vi "path steer2.vi"(11 "lane":bool) -> (3 "handle":dbl=5.200000000000001)   [LabVIEW 2015]
uses:
  G_ALL.vi
panel:
  in  "x 3":dbl=50.0 format="%#_13g"
  in  "x 2":dbl=5.0 format="%#_13g"
  in  "x":dbl=0.2 format="%#_13g"
  out "current idx":i32=9112
  out "map_track sel":dbl[][](array[numeric])
  out "dist sel":dbl[](array[numeric])
  in  "y":dbl=0.7
  in  "y 3":dbl=6.0 format="%#_13g"
  in  "y 2":dbl=15.0 format="%#_13g"
  out "element":dbl=-42.73390488941538
  out "XY Graph":cluster{"Y":dbl[], "Y":dbl[]}[](graph)=[{"Y"=[-62.270788198222405, -61.3028587435479, -60.64797168770746, -60.00414081408834, -59.35624672898274, -58.704182799096586, -58.062869555030055, -57.324417698249775, -56.3593175353864, -55.392505243639526, -54.74987553944367, -54.107360311157855, -53.4625281010745, -52.815268660483156, -51.84490266882976, -51.19638678084248, -50.22569981527318, -49.58323485281044, -48.93987198407685, -47.97817047579251, -47.33548315463016, -46.59804499224549, -45.95694180099581, -45.31659197029625, -44.3487464210446, -43.69981062781701, -42.73390488941538, -42.082599966834195, -41.437244759678, -40.79791938631003, -40.15638313566361, -39.5161574223998, -38.23493066806538, -37.59359481763489, -36.95200424827834, -36.31462462205997, -35.66938436512903, -34.97187443953064, -34.00375998116469, -33.361996827642564, -32.72011649020922, -31.762676240541964, -31.1267605203253, -30.48871011333479, -29.53221842324259, -28.8954579631871, -28.254818864117063, -27.61302081515921, -26.651631628034465, -25.91417367981147, -24.952481253026605, -24.309631425841772, -23.676791629873463], "Y"=[206.05300612625732, 206.20998608028694, 206.31731108964544, 206.4238193812488, 206.5319939554686, 206.64187408533144, 206.75094671337308, 206.84947177394332, 207.01722005802338, 207.18752464015114, 207.30187909576753, 207.4172264991964, 207.5340024404453, 207.6519836568955, 207.83122212678202, 207.95212683530963, 208.13494101670534, 208.25718613007166, 208.38030959441758, 208.56619920738456, 208.6915241088362, 208.80142519721795, 208.92844487701353, 209.05595576734015, 209.25069887260085, 209.3822220550732, 209.5796218846342, 209.7138886173675, 209.84754269369316, 209.98075087695668, 210.11518464043854, 210.24985120575727, 210.52176541203883, 210.65907131753448, 210.79696807600604, 210.9346992584219, 211.07492355438725, 211.2107438653489, 211.4245125721372, 211.5671731458532, 211.71064662911698, 211.92621966104974, 212.0703122033147, 212.2156875009412, 212.4352208971859, 212.58227341216255, 212.73101817081624, 212.88079472174562, 213.10672138794857, 213.28129607537733, 213.51073950832134, 213.66518203900827, 213.81774856058888]}, {"Y"=array[360 elements], "Y"=array[360 elements]}]
  out "map_track":dbl[][](array[numeric])=[[-62.270788198222405, 206.05300612625732], [-61.3028587435479, 206.20998608028694], [-60.64797168770746, 206.31731108964544], [-60.00414081408834, 206.4238193812488], [-59.35624672898274, 206.5319939554686], [-58.704182799096586, 206.64187408533144], [-58.062869555030055, 206.75094671337308], [-57.324417698249775, 206.84947177394332], [-56.3593175353864, 207.01722005802338], [-55.392505243639526, 207.18752464015114], [-54.74987553944367, 207.30187909576753], [-54.107360311157855, 207.4172264991964], [-53.4625281010745, 207.5340024404453], [-52.815268660483156, 207.6519836568955], [-51.84490266882976, 207.83122212678202], [-51.19638678084248, 207.95212683530963], [-50.22569981527318, 208.13494101670534], [-49.58323485281044, 208.25718613007166], [-48.93987198407685, 208.38030959441758], [-47.97817047579251, 208.56619920738456], [-47.33548315463016, 208.6915241088362], [-46.59804499224549, 208.80142519721795], [-45.95694180099581, 208.92844487701353], [-45.31659197029625, 209.05595576734015], [-44.3487464210446, 209.25069887260085], [-43.69981062781701, 209.3822220550732], [-42.73390488941538, 209.5796218846342], [-42.082599966834195, 209.7138886173675], [-41.437244759678, 209.84754269369316], [-40.79791938631003, 209.98075087695668], [-40.15638313566361, 210.11518464043854], [-39.5161574223998, 210.24985120575727], [-38.23493066806538, 210.52176541203883], [-37.59359481763489, 210.65907131753448], [-36.95200424827834, 210.79696807600604], [-36.31462462205997, 210.9346992584219], [-35.66938436512903, 211.07492355438725], [-34.97187443953064, 211.2107438653489], [-34.00375998116469, 211.4245125721372], [-33.361996827642564, 211.5671731458532], [-32.72011649020922, 211.71064662911698], [-31.762676240541964, 211.92621966104974], [-31.1267605203253, 212.0703122033147], [-30.48871011333479, 212.2156875009412], [-29.53221842324259, 212.4352208971859], [-28.8954579631871, 212.58227341216255], [-28.254818864117063, 212.73101817081624], [-27.61302081515921, 212.88079472174562], [-26.651631628034465, 213.10672138794857], [-25.91417367981147, 213.28129607537733], [-24.952481253026605, 213.51073950832134], [-24.309631425841772, 213.66518203900827], [-23.676791629873463, 213.81774856058888]]
  out "dist":dbl[](array[numeric])=[-20.832094988384732, -19.8553041899657, -18.874727759944605, -18.211104588592054, -17.558523398263937, -16.901660791573594, -16.240403646752558, -15.589881152775536, -14.844885627682299, -13.865315410117493, -12.883618074822659, -12.2308931111174, -11.578106130467432, -10.922785445885511, -10.264861171497461, -9.27808025010812, -8.61839031874266, -7.630638219294179, -6.976646555922144, -6.3216082606081, -5.342105968983386, -4.687313388290825, -3.941730869406446, -3.2881657992313187, -2.635243956437811, -1.648000377451759, -0.9858704723425199, 1.324050382980464, 1.977105781207095, 2.6325759923136727, 3.286811460402093, 4.596574542690249, 5.252443877774635, 5.9086861917571, 6.560777187390371, 7.221078514277543, 7.931688993516377, 8.923123643119611, 9.580551954444903, 10.238271505592612, 11.219680474262686, 11.871716872015202, 12.526119117620228, 13.507481061647026, 14.16100101214439, 14.81868137409002, 15.477724430966466, 16.465303302609627, 17.22314269645568, 18.211826980021506, 18.87296871643959, 19.523939338549425, 20.177455296801384]
  out "weight":dbl[](array[numeric])=[0.0, 0.0, 0.0, 0.0, 0.0, 0.0, 0.0, 0.0, 0.0, 0.0, 0.0, 0.0, 0.0, 0.0, 0.0, 0.0, 0.0, 0.0, 0.0, 0.0, 0.0, 0.0, 0.0, 0.0, 0.0, 0.0, 0.0, 0.006618568895935004, 0.022925143850115227, 0.045607515278417665, 0.07608403237613132, 0.16836029257577229, 0.23176392233689572, 0.30677978733130234, 0.39181799555917685, 0.48644996623238884, 0.5939963001932036, 0.7424840008349528, 0.8317946790700433, 0.9072191609257558, 0.9789386113637093, 0.9976924878056614, 1.0, 1.0, 1.0, 1.0, 1.0, 1.0, 1.0, 0.9944116041666606, 0.9486136733425102, 0.8544723463308531, 0.7254699057656591]
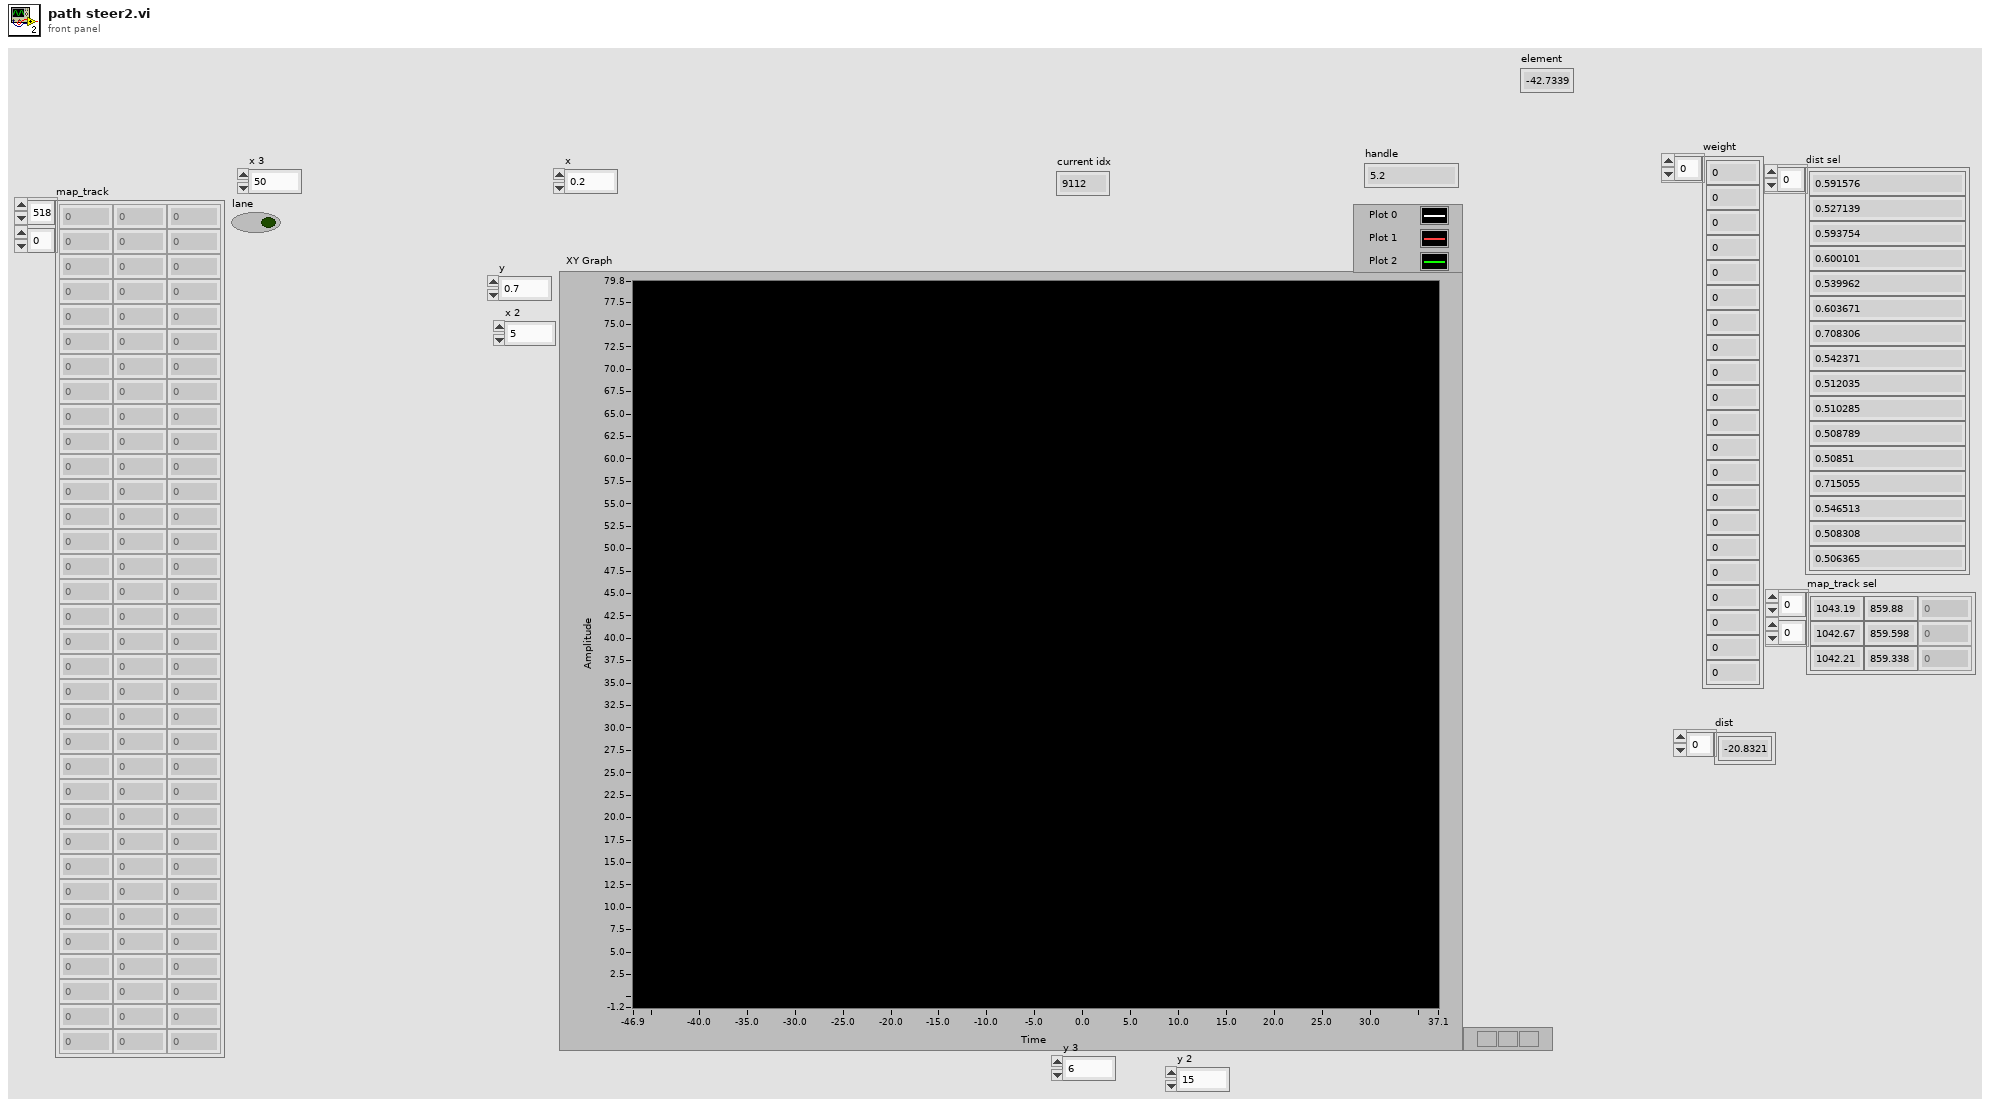
[diagram p1: front panel]
types:
  T1 = cluster{"Steer_input":dbl, "Steer_output":dbl, "VS_des":dbl, "VS_can":dbl, "heading":dbl, "auto":bool, "run":bool, "x":dbl, "y":dbl}
  T2 = cluster{"C_Wheel base":dbl, "ratio_steer":dbl, "Overall width":dbl, "af":dbl, "turn radius":dbl, "eval":dbl, "ap":dbl, "an":dbl, "Vmax":dbl, "mu":dbl, "Vlast":dbl}
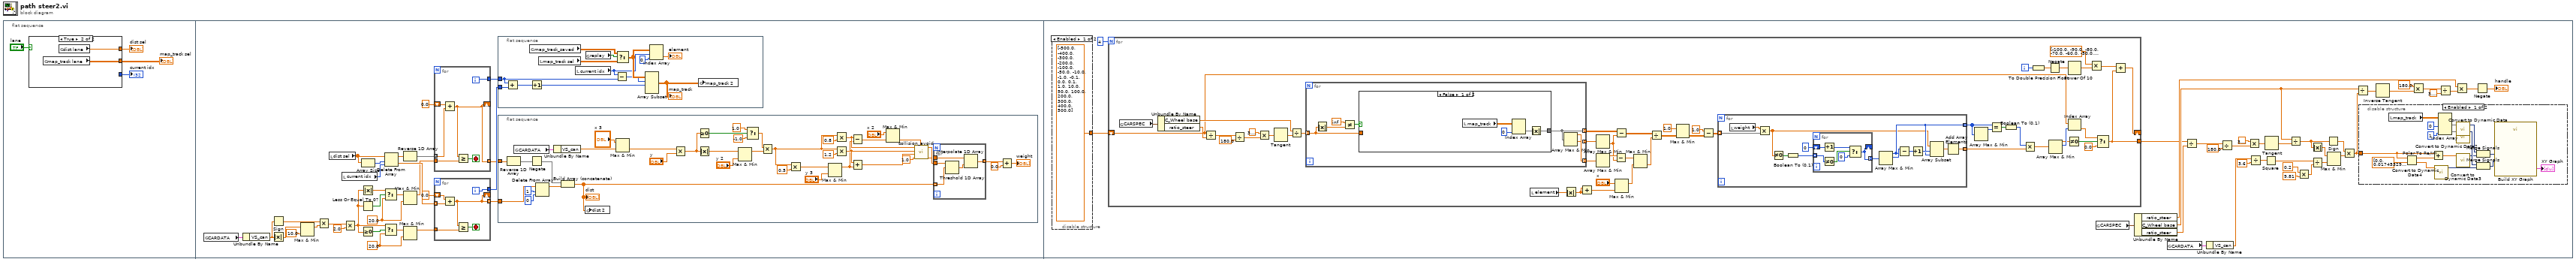
[diagram p0: block diagram]
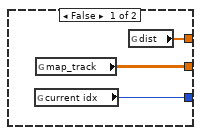
[diagram p2: hidden frame]
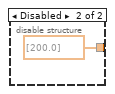
[diagram p3: hidden frame]
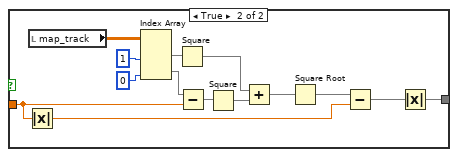
[diagram p5: hidden frame]
diagram:
  n1 = flat-sequence {
    frame #0 {
      n2 = case shown="True" "lane" {
        tunnel: [w7 _] -> w3
        tunnel: [w6 w9] -> w2
        tunnel: [w5 w8] -> w1
        frame False {
          n3 = global read "G_ALL.vi" "current idx"() -> (w7:i32)
          n4 = global read "G_ALL.vi" "map_track"() -> (w5:dbl[][])
          n5 = global read "G_ALL.vi" "dist"() -> (w6:dbl[])
        }
        frame True {
          n6 = global read "G_ALL.vi" "map_track lane"() -> (w8:dbl[][])
          n7 = global read "G_ALL.vi" "dist lane"() -> (w9:dbl[])
        }
      }
      "dist sel" <- w2
      "map_track sel" <- w1
      "current idx" <- w3
    }
    frame #1 {
      w25 = 20.0 ("y")
      w27 = 20.0 ("y")
      n8 = global read "G_ALL.vi" "CARDATA"() -> (w14:T1)
      n9 = Unbundle By Name(w14) -> ("VS_can"=w17:dbl)
      n10 = Sign(1:w17) -> (0:w18:dbl)
      n11 = Absolute Value(x=w17) -> (abs(x)=w15:dbl)
      n12 = Max & Min(x=w15, y=10.0) -> (max(x,y)=w19:dbl)  [unwired: 1 out]
      n13 = Multiply(x=w18, y=w19) -> (x*y=w13:dbl)
      n14 = local read "dist sel"() -> (w11:dbl[])
      n15 = local read "current idx"() -> (w10:i32)
      n16 = Multiply(x=w13, y=2.0) -> (x*y=w12:dbl)
      n17 = Array Size(array=w11) -> (size(s)=w39:i32)
      n18 = Absolute Value(x=w12) -> (abs(x)=w21:dbl)
      n19 = Less Or Equal To 0?(x=w12) -> (x <= 0?=w23:bool)
      n20 = Greater Or Equal To 0?(x=w12) -> (x >= 0?=w29:bool)
      n21 = Select(t=w21, s=w23, f=w25) -> (s? t:f=w24:dbl)
      n22 = Select(t=w12, s=w29, f=w27) -> (s? t:f=w28:dbl)
      n23 = Delete From Array(array=w11, length=w39, index=w10) -> (deleted portion=w35:dbl[], array with subset deleted=w38:dbl[])
      n24 = Reverse 1D Array(array=w38) -> (reversed array=w37:dbl[])
      n25 = Max & Min(x=w24, y=w25) -> (max(x,y)=w20:dbl)  [unwired: 1 out]
      n26 = Max & Min(x=w28, y=w27) -> (max(x,y)=w26:dbl)  [unwired: 1 out]
      n27 = for {
        tunnel: w37 -> [w108] mode=indexing
        shift-right: [w105] -> _
        shift-left: 0.0 -> [w109]
        tunnel: [w106] -> w33
        tunnel: [w105] -> w31 mode=indexing
        tunnel: w20 -> [w104]
        i -> [w106]
        stop <- w107 stop-if-true
        n28 = Add(x=w109, y=w108) -> (x+y=w105:dbl)
        n29 = Greater Or Equal?(x=w105, y=w104) -> (x >= y?=w107:bool)
      }
      n30 = for {
        tunnel: w35 -> [w102] mode=indexing
        shift-right: [w99] -> _
        shift-left: 0.0 -> [w103]
        tunnel: [w100] -> w32
        tunnel: [w99] -> w30 mode=indexing
        tunnel: w26 -> [w98]
        i -> [w100]
        stop <- w101 stop-if-true
        n31 = Add(x=w103, y=w102) -> (x+y=w99:dbl)
        n32 = Greater Or Equal?(x=w99, y=w98) -> (x >= y?=w101:bool)
      }
      n33 = flat-sequence {
        tunnel: w33 -> [w48]
        tunnel: w32 -> [w47]
        frame #0 {
          n34 = Add(x=w48, y=w47) -> (x+y=w46:i32)
          n35 = global read "G_ALL.vi" "map_track_saved"() -> (w50:dbl[][])
          n36 = Increment(x=w46) -> (x+1=w44:i32)
          n37 = local read "map_track sel"() -> (w41:dbl[][])
          n38 = local read "current idx"() -> (w40:i32)
          n39 = global read "G_ALL.vi" "replay"() -> (w51:bool)
          n40 = Subtract(x=w40, y=w48) -> (x-y=w45:i32)
          n41 = Select(t=w50, s=w51, f=w41) -> (s? t:f=w52:dbl[][])
          n42 = Array Subset(array=w52, index (row)=w45, length (row)=w44) -> (w49:dbl[][])  [unwired: 2 in]
          "map_track" <- w49
          n43 = Index Array(array=w52, index (row)=w40, index (col)=0 ("disabled index (col)")) -> (element=→"element":dbl)
          n44 = global write "G_ALL.vi" "map_track 2"(w49) -> ()
        }
      }
      n45 = flat-sequence {
        tunnel: w31 -> [w85]
        tunnel: w30 -> [w83]
        frame #0 {
          n46 = Reverse 1D Array(array=w85) -> (reversed array=w84:dbl[])
          n47 = global read "G_ALL.vi" "CARDATA"() -> (w89:T1)
          n48 = Negate(x=w84) -> (-x=w80:dbl[])
          n49 = Delete From Array(array=w83, length=1, index=0) -> (array with subset deleted=w79:dbl[])  [unwired: 1 out]
          n50 = Unbundle By Name(w89) -> ("VS_can"=w55:dbl)
          n51 = Build Array (concatenate)(w80, w79) -> (w91:dbl[])
          "dist" <- w91
          n52 = global write "G_ALL.vi" "dist 2"(w91) -> ()
          n53 = Max & Min(x="x 3", y=w55) -> (min(x,y)=w53:dbl)  [unwired: 1 out]
          n54 = Multiply(x=w53, y="y") -> (x*y=w60:dbl)
          n55 = Greater Or Equal To 0?(x=w60) -> (x >= 0?=w67:bool)
          n56 = Absolute Value(x=w60) -> (abs(x)=w73:dbl)
          n57 = Max & Min(x=w73, y="y 2") -> (max(x,y)=w71:dbl)  [unwired: 1 out]
          n58 = Select(t=1.0, s=w67, f=-1.0) -> (s? t:f=w66:dbl)
          n59 = Multiply(x=w66, y=w71) -> (x*y=w69:dbl)
          n60 = Multiply(x=w69, y=0.5) -> (x*y=w63:dbl)
          n61 = Max & Min(x=w63, y="y 3") -> (max(x,y)=w62:dbl)  [unwired: 1 out]
          n62 = Multiply(x=w69, y=0.8) -> (x*y=w75:dbl)
          n63 = Multiply(x=w69, y=1.2) -> (x*y=w68:dbl)
          n64 = Subtract(x=w75, y=w62) -> (x-y=w58:dbl)
          n65 = Add(x=w68, y=w62) -> (x+y=w78:dbl)
          n66 = Max & Min(x="x 2", y=w58) -> (min(x,y)=w57:dbl)  [unwired: 1 out]
          n67 = call "collision_avoid.vi"("x0"=w57, "d"=1.0, "x3"=w78, "x2"=w68, "x1"=w75) -> ("y"=w86:dbl[], "x"=w87:dbl[])  [unwired: 5 in]
          n68 = for {
            tunnel: w91 -> [w96] mode=indexing
            tunnel: w87 -> [w97]
            tunnel: w86 -> [w95]
            tunnel: [w93] -> w77 mode=indexing
            n69 = Threshold 1D Array(2:w96, 3:w97) -> (0:w94:dbl)  [unwired: 1 in]
            n70 = Interpolate 1D Array(1:w94, 2:w95) -> (0:w93:dbl)
          }
          n71 = Add(x=w77, y=0.0 ("d")) -> (x+y=→"weight":dbl[])
        }
      }
    }
    frame #2 {
      n72 = disable-structure shown="Enabled" {
        disable-tunnel: [dbl[] [-500.0, -400.0, -300.0, -200.0, -100.0, -50.0, -10.0, -1.0, -0.1, 0.0, 0.1, 1.0, 10.0, 50.0, 100.0, 200.0, 300.0, 400.0, 500.0] ("theta") dbl[] [200.0] ("theta")] -> w110
        frame Enabled {
        }
        frame Disabled {
        }
      }
      n73 = for {
        N: 4 -> [_]
        tunnel: [w177] -> w111
        shift-right: [w196] -> _
        shift-left: w110 -> [w197]
        i -> [w201]
        n74 = global read "G_ALL.vi" "CARSPEC"() -> (w203:T2)
        n75 = Unbundle By Name(w203) -> ("C_Wheel base"=w211:dbl, "ratio_steer"=w209:dbl)
        n76 = Divide(x=w197, y=w209) -> (x/y=w208:dbl[])
        n77 = Divide(x=w208, y=180.0) -> (x/y=w205:dbl[])
        n78 = Multiply(x=3.141592653589793, y=w205) -> (x*y=w207:dbl[])
        n79 = Tangent(1:w207) -> (0:w210:dbl[])
        n80 = Divide(x=w211, y=w210) -> (x/y=w202:dbl[])
        n81 = for {
          tunnel: w202 -> [w237] mode=indexing
          tunnel: [w233] -> w193 mode=indexing
          tunnel: [w232] -> w194 mode=indexing
          tunnel: [w231] -> w192 mode=indexing
          n82 = Absolute Value(x=w237) -> (abs(x)=w235:dbl)
          n83 = Not Equal?(x=inf, y=w235) -> (x != y?=w234:bool)
          n84 = case shown="False" w234 {
            tunnel: w237 -> [_ w255]
            tunnel: [w239 w254] -> w231
            frame False {
              n85 = local read "map_track"() -> (w238:dbl[][])
              n86 = Index Array(array=w238, index (col)=0) -> (element=w240:dbl[])  [unwired: 1 in]
              n87 = Absolute Value(x=w240) -> (abs(x)=w239:dbl[])
            }
            frame True {
              n88 = Absolute Value(x=w255) -> (abs(x)=w245:dbl)
              n89 = local read "map_track"() -> (w251:dbl[][])
              n90 = Index Array(array=w251, index (col) #1=1 ("disabled index (col)"), index (col) #2=0 ("disabled index (col)")) -> (element #1=w248:dbl[], element #2=w250:dbl[])  [unwired: 2 in]
              n91 = Square(x=w248) -> (x^2=w247:dbl[])
              n92 = Subtract(x=w250, y=w255) -> (x-y=w249:dbl[])
              n93 = Square(x=w249) -> (x^2=w246:dbl[])
              n94 = Add(x=w247, y=w246) -> (x+y=w242:dbl[])
              n95 = Square Root(x=w242) -> (sqrt(x)=w244:dbl[])
              n96 = Subtract(x=w244, y=w245) -> (x-y=w243:dbl[])
              n97 = Absolute Value(x=w243) -> (abs(x)=w254:dbl[])
            }
          }
          n98 = Array Max & Min(array=w231) -> (max value=w233:dbl, min value=w232:dbl)  [unwired: 2 out]
        }
        n99 = local read "element"() -> (w183:dbl)
        n100 = Absolute Value(x=w183) -> (abs(x)=w164:dbl)
        n101 = Add(x=w164, y=w164) -> (x+y=w175:dbl)
        n102 = Array Max & Min(array=w194) -> (min value=w190:dbl)  [unwired: 3 out]
        n103 = Array Max & Min(array=w193) -> (max value=w191:dbl)  [unwired: 3 out]
        n104 = Subtract(x=w191, y=w190) -> (x-y=w187:dbl)
        n105 = Subtract(x=w192, y=w190) -> (x-y=w185:dbl[][])
        n106 = Max & Min(x="x", y=w175) -> (max(x,y)=w181:dbl)  [unwired: 1 out]
        n107 = Max & Min(x=w187, y=w181) -> (min(x,y)=w186:dbl)  [unwired: 1 out]
        n108 = Divide(x=w185, y=w186) -> (x/y=w184:dbl[][])
        n109 = Max & Min(x=1.0 ("y"), y=w184) -> (min(x,y)=w172:dbl[][])  [unwired: 1 out]
        n110 = Subtract(x=1.0 ("y"), y=w172) -> (x-y=w170:dbl[][])
        n111 = for {
          tunnel: w170 -> [w216] mode=indexing
          tunnel: [w215] -> w171 mode=indexing
          tunnel: [w217] -> w169 mode=indexing
          n112 = local read "weight"() -> (w218:dbl[])
          n113 = Multiply(x=w218, y=w216) -> (x*y=w212:dbl[])
          n114 = Not Equal To 0?(x=w212) -> (x != 0?=w214:bool[])
          n115 = Boolean To (0,1)(Boolean=w214) -> (0, 1=w213:i16[])
          n116 = for {
            tunnel: w213 -> [w230] mode=indexing
            shift-right: [w225] -> _
            shift-left: 0 -> [w228]
            tunnel: [w225] -> w223 mode=indexing
            n117 = Increment(x=w228) -> (x+1=w227:i32)
            n118 = Not Equal To 0?(x=w230) -> (x != 0?=w229:bool)
            n119 = Select(t=w227, s=w229, f=0) -> (s? t:f=w225:i32)
          }
          n120 = Array Max & Min(array=w223) -> (max value=w217:i32, max index (indices)=w222:i32)  [unwired: 2 out]
          n121 = Subtract(x=w222, y=w217) -> (x-y=w221:i32)
          n122 = Increment(x=w221) -> (x+1=w220:i32)
          n123 = Array Subset(array=w212, index=w220, length=w217) -> (w219:dbl[])
          n124 = Add Array Elements(numeric array=w219) -> (sum=w215:dbl)
        }
        n125 = Array Max & Min(array=w169) -> (max value=w166:i32)  [unwired: 3 out]
        n126 = Equal?(x=w169, y=w166) -> (x = y?=w168:bool[])
        n127 = Boolean To (0,1)(Boolean=w168) -> (0, 1=w167:i16[])
        n128 = Multiply(x=w167, y=w171) -> (x*y=w165:dbl[])
        n129 = To Double Precision Float(number=w201) -> (double precision float=w199:dbl)
        n130 = Negate(x=w199) -> (-x=w198:dbl)
        n131 = Array Max & Min(array=w165) -> (max value=w180:dbl, max index (indices)=w189:i32)  [unwired: 2 out]
        n132 = Not Equal To 0?(x=w180) -> (x != 0?=w179:bool)
        n133 = Power Of 10(x=w198) -> (10^x=w188:dbl)
        n134 = Index Array(array=w197, index=w189) -> (element=w178:dbl)
        n135 = Multiply(x=dbl[] [-100.0, -90.0, -80.0, -70.0, -60.0, -50.0, -40.0, -30.0, -20.0, -10.0, 0.0, 10.0, 20.0, 30.0, 40.0, 50.0, 60.0, 70.0, 80.0, 90.0, 100.0], y=w188) -> (x*y=w195:dbl[])
        n136 = Select(t=w178, s=w179, f=0.0 ("handle")) -> (s? t:f=w177:dbl)
        n137 = Add(x=w195, y=w177) -> (x+y=w196:dbl[])
      }
      n138 = global read "G_ALL.vi" "CARSPEC"() -> (w117:T2)
      n139 = Unbundle By Name(w117) -> ("ratio_steer"=w115:dbl, "C_Wheel base"=w116:dbl, "ratio_steer"=w123:dbl)
      n140 = global read "G_ALL.vi" "CARDATA"() -> (w142:T1)
      n141 = Divide(x=w111, y=w123) -> (x/y=w122:dbl)
      n142 = Unbundle By Name(w142) -> ("VS_can"=w125:dbl)
      n143 = Divide(x=w122, y=180.0) -> (x/y=w119:dbl)
      n144 = Multiply(x=3.141592653589793, y=w119) -> (x*y=w121:dbl)
      n145 = Divide(x=w125, y=3.6) -> (x/y=w129:dbl)
      n146 = Square(x=w129) -> (x^2=w130:dbl)
      n147 = Tangent(1:w121) -> (0:w124:dbl)
      n148 = Divide(x=w116, y=w124) -> (x/y=w112:dbl)
      n149 = Multiply(x=0.2, y=9.81) -> (x*y=w131:dbl)
      n150 = Absolute Value(x=w112) -> (abs(x)=w132:dbl)
      n151 = Divide(x=w130, y=w131) -> (x/y=w133:dbl)
      n152 = Sign(1:w112) -> (0:w135:dbl)
      n153 = Max & Min(x=w132, y=w133) -> (max(x,y)=w134:dbl)  [unwired: 1 out]
      n154 = Multiply(x=w135, y=w134) -> (x*y=w143:dbl)
      n155 = Divide(x=w116, y=w143) -> (x/y=w141:dbl)
      n156 = disable-structure shown="Enabled" {
        disable-tunnel: w143 -> [w152 _]
        frame Enabled {
          n157 = local read "map_track"() -> (w149:dbl[][])
          n158 = Polar To Re/Im(2:dbl[] [0.0, 0.017453292519943295, 0.03490658503988659, 0.05235987755982988, 0.06981317007977318, 0.08726646259971647, 0.10471975511965977, 0.12217304763960307, 0.13962634015954636, 0.15707963267948966, 0.17453292519943295, 0.19198621771937624, 0.20943951023931953, 0.22689280275926282, 0.24434609527920614, 0.2617993877991494, 0.2792526803190927, 0.296705972839036, 0.3141592653589793, 0.33161255787892263, 0.3490658503988659, 0.3665191429188092, 0.3839724354387525, 0.40142572795869574, 0.41887902047863906, 0.4363323129985824, 0.45378560551852565, 0.47123889803846897, 0.4886921905584123, 0.5061454830783556, 0.5235987755982988, 0.5410520681182421, 0.5585053606381855, 0.5759586531581287, 0.593411945678072, 0.6108652381980153, 0.6283185307179586, 0.6457718232379019, 0.6632251157578453, 0.6806784082777886, 0.6981317007977318, 0.7155849933176751, 0.7330382858376184, 0.7504915783575618, 0.767944870877505, 0.7853981633974483, 0.8028514559173915, 0.8203047484373349, 0.8377580409572781, 0.8552113334772213, 0.8726646259971648, 0.890117918517108, 0.9075712110370513, 0.9250245035569946, 0.9424777960769379, 0.9599310885968813, 0.9773843811168246, 0.9948376736367678, 1.0122909661567112, 1.0297442586766543, 1.0471975511965976, 1.064650843716541, 1.0821041362364843, 1.0995574287564276, 1.117010721276371, 1.1344640137963142, 1.1519173063162573, 1.1693705988362009, 1.186823891356144, 1.2042771838760875, 1.2217304763960306, 1.239183768915974, 1.2566370614359172, 1.2740903539558606, 1.2915436464758039, 1.3089969389957472, 1.3264502315156905, 1.3439035240356336, 1.3613568165555772, 1.3788101090755203, 1.3962634015954636, 1.413716694115407, 1.4311699866353502, 1.4486232791552935, 1.4660765716752369, 1.48352986419518, 1.5009831567151235, 1.5184364492350666, 1.53588974175501, 1.5533430342749532, 1.5707963267948966, 1.5882496193148399, 1.605702911834783, 1.6231562043547265, 1.6406094968746698, 1.6580627893946132, 1.6755160819145563, 1.6929693744344996, 1.7104226669544427, 1.7278759594743864, 1.7453292519943295, 1.7627825445142729, 1.780235837034216, 1.7976891295541593, 1.8151424220741026, 1.8325957145940461, 1.8500490071139892, 1.8675022996339325, 1.8849555921538759, 1.902408884673819, 1.9198621771937625, 1.9373154697137058, 1.9547687622336491, 1.9722220547535922, 1.9896753472735356, 2.007128639793479, 2.0245819323134224, 2.0420352248333655, 2.0594885173533086, 2.076941809873252, 2.0943951023931953, 2.111848394913139, 2.129301687433082, 2.1467549799530254, 2.1642082724729685, 2.1816615649929116, 2.199114857512855, 2.2165681500327987, 2.234021442552742, 2.251474735072685, 2.2689280275926285, 2.2863813201125716, 2.3038346126325147, 2.321287905152458, 2.3387411976724017, 2.356194490192345, 2.373647782712288, 2.3911010752322315, 2.408554367752175, 2.426007660272118, 2.443460952792061, 2.4609142453120048, 2.478367537831948, 2.495820830351891, 2.5132741228718345, 2.530727415391778, 2.548180707911721, 2.5656340004316642, 2.5830872929516078, 2.600540585471551, 2.6179938779914944, 2.6354471705114375, 2.652900463031381, 2.670353755551324, 2.6878070480712672, 2.705260340591211, 2.7227136331111543, 2.7401669256310974, 2.7576202181510405, 2.7750735106709836, 2.792526803190927, 2.8099800957108707, 2.827433388230814, 2.844886680750757, 2.8623399732707004, 2.8797932657906435, 2.897246558310587, 2.91469985083053, 2.9321531433504737, 2.949606435870417, 2.96705972839036, 2.9845130209103035, 3.001966313430247, 3.01941960595019, 3.036872898470133, 3.0543261909900767, 3.07177948351002, 3.089232776029963, 3.1066860685499065, 3.12413936106985, 3.141592653589793, 3.159045946109736, 3.1764992386296798, 3.193952531149623, 3.211405823669566, 3.2288591161895095, 3.246312408709453, 3.2637657012293966, 3.2812189937493397, 3.2986722862692828, 3.3161255787892263, 3.3335788713091694, 3.3510321638291125, 3.368485456349056, 3.385938748868999, 3.4033920413889422, 3.4208453339088853, 3.4382986264288293, 3.455751918948773, 3.473205211468716, 3.490658503988659, 3.5081117965086026, 3.5255650890285457, 3.543018381548489, 3.560471674068432, 3.5779249665883754, 3.5953782591083185, 3.6128315516282616, 3.630284844148205, 3.647738136668149, 3.6651914291880923, 3.6826447217080354, 3.7000980142279785, 3.717551306747922, 3.735004599267865, 3.752457891787808, 3.7699111843077517, 3.787364476827695, 3.804817769347638, 3.8222710618675815, 3.839724354387525, 3.8571776469074686, 3.8746309394274117, 3.8920842319473548, 3.9095375244672983, 3.9269908169872414, 3.9444441095071845, 3.961897402027128, 3.979350694547071, 3.9968039870670142, 4.014257279586958, 4.031710572106902, 4.049163864626845, 4.066617157146788, 4.084070449666731, 4.101523742186674, 4.118977034706617, 4.136430327226561, 4.153883619746504, 4.171336912266447, 4.1887902047863905, 4.206243497306334, 4.223696789826278, 4.241150082346221, 4.258603374866164, 4.276056667386108, 4.293509959906051, 4.310963252425994, 4.328416544945937, 4.34586983746588, 4.363323129985823, 4.380776422505767, 4.39822971502571, 4.4156830075456535, 4.4331363000655974, 4.4505895925855405, 4.468042885105484, 4.485496177625427, 4.50294947014537, 4.520402762665314, 4.537856055185257, 4.5553093477052, 4.572762640225143, 4.590215932745086, 4.607669225265029, 4.625122517784973, 4.642575810304916, 4.66002910282486, 4.6774823953448035, 4.694935687864747, 4.71238898038469, 4.729842272904633, 4.747295565424576, 4.764748857944519, 4.782202150464463, 4.799655442984406, 4.81710873550435, 4.834562028024293, 4.852015320544236, 4.869468613064179, 4.886921905584122, 4.9043751981040655, 4.9218284906240095, 4.939281783143953, 4.956735075663896, 4.974188368183839, 4.991641660703782, 5.009094953223726, 5.026548245743669, 5.044001538263612, 5.061454830783556, 5.078908123303499, 5.096361415823442, 5.113814708343385, 5.1312680008633285, 5.148721293383272, 5.1661745859032155, 5.183627878423159, 5.201081170943102, 5.218534463463046, 5.235987755982989, 5.253441048502932, 5.270894341022875, 5.288347633542818, 5.305800926062762, 5.323254218582705, 5.340707511102648, 5.358160803622591, 5.3756140961425345, 5.393067388662478, 5.410520681182422, 5.427973973702365, 5.445427266222309, 5.462880558742252, 5.480333851262195, 5.497787143782138, 5.515240436302081, 5.532693728822024, 5.550147021341967, 5.567600313861911, 5.585053606381854, 5.602506898901798, 5.619960191421741, 5.6374134839416845, 5.654866776461628, 5.672320068981571, 5.689773361501514, 5.707226654021458, 5.724679946541401, 5.742133239061344, 5.759586531581287, 5.77703982410123, 5.794493116621174, 5.811946409141117, 5.82939970166106, 5.846852994181004, 5.8643062867009474, 5.8817595792208905, 5.899212871740834, 5.916666164260777, 5.93411945678072, 5.951572749300664, 5.969026041820607, 5.98647933434055, 6.003932626860494, 6.021385919380437, 6.03883921190038, 6.056292504420323, 6.073745796940266, 6.09119908946021, 6.1086523819801535, 6.126105674500097, 6.14355896702004, 6.161012259539983, 6.178465552059926, 6.19591884457987, 6.213372137099813, 6.230825429619757, 6.2482787221397, 6.265732014659643] ("x*y"), 3:w152) -> (0:w155:dbl[], 1:w151:dbl[])
          n159 = Add(x=w152, y=w151) -> (x+y=w150:dbl[])
          n160 = call "Convert to Dynamic Data4"("Array"=w155) -> ("Dynamic Data Type"=w154:dynamicdata)  [unwired: 3 in]
          n161 = Index Array(array=w149, index (col) #1=0 ("disabled index (col)"), index (col) #2=1 ("disabled index (col)")) -> (element #1=w148:dbl[], element #2=w147:dbl[])  [unwired: 2 in]
          n162 = call "Convert to Dynamic Data"("Array"=w148) -> ("Dynamic Data Type"=w160:dynamicdata)  [unwired: 3 in]
          n163 = call "Convert to Dynamic Data2"("Array"=w147) -> ("Dynamic Data Type"=w159:dynamicdata)  [unwired: 3 in]
          n164 = call "Convert to Dynamic Data3"("Array"=w150) -> ("Dynamic Data Type"=w157:dynamicdata)  [unwired: 3 in]
          n165 = Merge Signals(w160, w157) -> (w158:dynamicdata)
          n166 = Merge Signals(w159, w154) -> (w156:dynamicdata)
          n167 = call "Build XY Graph"("Y Input"=w156, "X Input"=w158) -> ("XY Graph"=→"XY Graph":cluster{"X":dbl[], "Y":dbl[]}[])  [unwired: 8 in, 1 out]
        }
        frame Disabled {
        }
      }
      n168 = Inverse Tangent(1:w141) -> (0:w139:dbl)
      n169 = Multiply(x=180.0 ("y"), y=w139) -> (x*y=w138:dbl)
      n170 = Divide(x=w138, y=3.141592653589793) -> (x/y=w136:dbl)
      n171 = Multiply(x=w115, y=w136) -> (x*y=w113:dbl)
      n172 = Negate(x=w113) -> (-x=→"handle":dbl)
    }
  }
